vi "Yogurt cup query.vi"() -> (3 "Enum":T1)   [LabVIEW 2020]
uses:
  Estados.ctl
  Variables Globales.vi
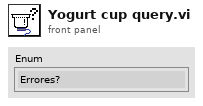
[diagram p1: front panel]
types:
  T1 = typedef "Estados.ctl" = enum16{"Errores?", "Control de válvula alt.", "Control de válvula", "Nivel bajo?", "Query nivel del tanque", "Query peso del pote", "Ajuste?", "Llenado?", "Emergencia?", "Init", "Ajuste", "Nivel Bajo", "Llenado", "Error", "Emergencia"}
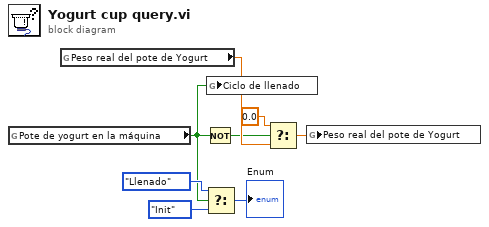
[diagram p0: block diagram]
diagram:
  n1 = global read "Variables Globales.vi" "Pote de yogurt en la máquina"() -> (w1:bool)
  n2 = global read "Variables Globales.vi" "Peso real del pote de Yogurt"() -> (w5:dbl)
  n3 = Not(x=w1) -> (.not. x?=w3:bool)
  n4 = Select(t=Estados."Llenado", s=w1, f=Estados."Init") -> (s? t:f=→"Enum":T1)
  n5 = global write "Variables Globales.vi" "Ciclo de llenado"(w1) -> ()
  n6 = Select(t=0.0, s=w3, f=w5) -> (s? t:f=w4:dbl)
  n7 = global write "Variables Globales.vi" "Peso real del pote de Yogurt"(w4) -> ()
